vi "ScaleTo32Bit_x410.vi"(8 "valid in":bool, 10 "factor":u16, 11 "val":fxp<+/-,18,1>) -> (0 "valid out":bool, 3 "32 bit fxp":fxp<+/-,32,14>)   [LabVIEW 2025]
uses:
  <vilib>/rvi/FXPMathLib/FxpConvert/subVIs/nifxpmath_Convert_SimConfig.ctl
  <vilib>/fxp/LVFixedPointQuantizationPolicyTypeDef.ctl
  <vilib>/fxp/LVFixedPointOverflowPolicyTypeDef.ctl
  <vilib>/rvi/FXPMathLib/FxpConvert/simVIs/DllFxpConvertTemp_sub.vi
  <vilib>/rvi/FXPMathLib/FxpInterpret/XNode/nifxpmath_Interpret.xnode
  <vilib>/rvi/FXPMathLib/FxpConvert/XNode/nifxpmath_Convert.xnode
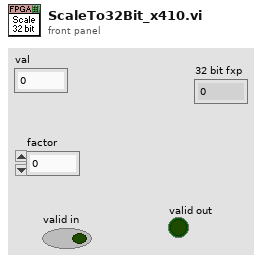
[diagram p1: front panel]
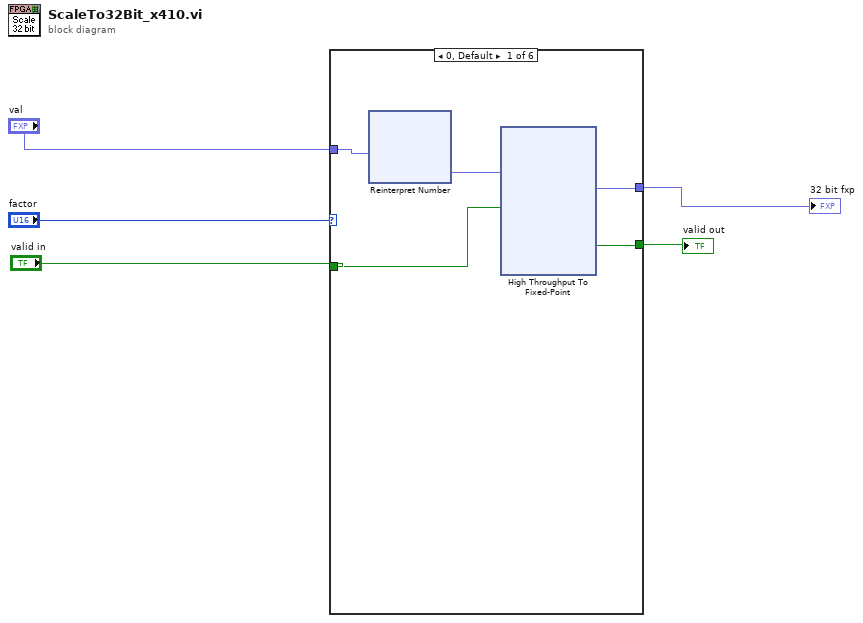
[diagram p0: block diagram]
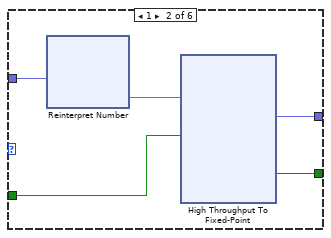
[diagram p2: hidden frame]
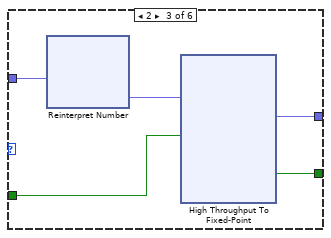
[diagram p3: hidden frame]
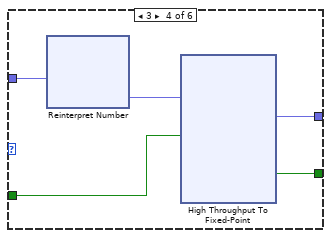
[diagram p4: hidden frame]
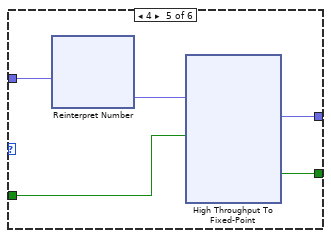
[diagram p5: hidden frame]
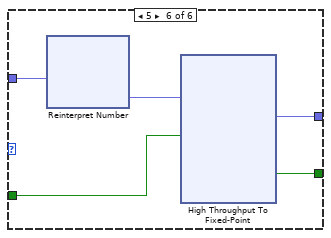
[diagram p6: hidden frame]
diagram:
  n1 = case shown="0, Default" "factor" {
    tunnel: "valid in" -> [w10 w37 w66 w95 w122 w153]
    tunnel: "val" -> [w7 w38 w67 w96 w125 w154]
    tunnel: [w8 w36 w64 w93 w123 w151] -> w3
    tunnel: [w9 w35 w65 w94 w124 w152] -> w1
    frame 0, Default {
      n2 = xnode "Reinterpret Number"("x"=w7) -> ("y"=w6:fxp<+/-,18,14>)
      n3 = xnode "High Throughput To Fixed-Point"("x"=w6, "input valid"=w10) -> ("y"=w9:fxp<+/-,32,14>, "output valid"=w8:bool)  [unwired: 1 in, 1 out]
    }
    frame 1 {
      n4 = xnode "Reinterpret Number"("x"=w38) -> ("y"=w39:fxp<+/-,18,15>)
      n5 = xnode "High Throughput To Fixed-Point"("x"=w39, "input valid"=w37) -> ("y"=w35:fxp<+/-,32,14>, "output valid"=w36:bool)  [unwired: 1 in, 1 out]
    }
    frame 2 {
      n6 = xnode "Reinterpret Number"("x"=w67) -> ("y"=w68:fxp<+/-,18,16>)
      n7 = xnode "High Throughput To Fixed-Point"("x"=w68, "input valid"=w66) -> ("y"=w65:fxp<+/-,32,14>, "output valid"=w64:bool)  [unwired: 1 in, 1 out]
    }
    frame 3 {
      n8 = xnode "Reinterpret Number"("x"=w96) -> ("y"=w97:fxp<+/-,18,17>)
      n9 = xnode "High Throughput To Fixed-Point"("x"=w97, "input valid"=w95) -> ("y"=w94:fxp<+/-,32,14>, "output valid"=w93:bool)  [unwired: 1 in, 1 out]
    }
    frame 4 {
      n10 = xnode "Reinterpret Number"("x"=w125) -> ("y"=w126:fxp<+/-,18,18>)
      n11 = xnode "High Throughput To Fixed-Point"("x"=w126, "input valid"=w122) -> ("y"=w124:fxp<+/-,32,14>, "output valid"=w123:bool)  [unwired: 1 in, 1 out]
    }
    frame 5 {
      n12 = xnode "Reinterpret Number"("x"=w154) -> ("y"=w155:fxp<+/-,18,19>)
      n13 = xnode "High Throughput To Fixed-Point"("x"=w155, "input valid"=w153) -> ("y"=w152:fxp<+/-,32,14>, "output valid"=w151:bool)  [unwired: 1 in, 1 out]
    }
  }
  "valid out" <- w3
  "32 bit fxp" <- w1
